vi "OAT FIR Preprocess Filter (N Channels).vi"(0 "scaled signals [EU]":waveform(dbl)[](array[waveform]), 1 "filter type":T3(ring), 2 "reset? (F)":bool, 5 "freq specs [Hz]":T2={"fpass 1"=100.0, "fstop 1"=200.0, "fpass 2"=0.0, "fstop 2"=0.0} {"fstop 2" format="%#.2f"; "fpass 2" format="%#.3f"; "fstop 1" format="%#.2f"; "fpass 1" format="%#.3f"}, 7 "ripple specs [dB]":T1={"passband ripple"=0.1, "stopband attenuation"=60.0} {"stopband attenuation" format="%#.2f"; "passband ripple" format="%#.2f"}, 11 "error in (no error)":errorcluster) -> (4 "filtered scaled signals [EU]":waveform(dbl)[](array[waveform]), 8 "taps":i32, 15 "error out":errorcluster)   [LabVIEW 2017, in "SoundVib_RefDataProcess.lvlib"]
doc: "Designs an FIR filter and filters the <B>scaled signal [EU]</B>. Wire data to the <B>scaled signal [EU]</B> input to determine the polymorphic instance to use or manually select the instance."
uses:
  <vilib>/addons/Sound and Vibration/Order Analysis/Referece Data Processing/SoundVib_RefDataProcess.lvlib
  <vilib>/addons/_NISVFA/_Shared subVIs/Common/svc_Check for Waveform Parameter Continuity (no state).vi
  <vilib>/addons/_NISVFA/_Shared subVIs/Common/svc_Get SV Channel Info.vi
  <vilib>/addons/_NISVFA/_Shared subVIs/Common/svc_Engineering Units to Unit Label.vi
  <vilib>/addons/_NISVFA/_Shared subVIs/Common/svc_Unit Label to Engineering Units.vi
  <vilib>/measure/NI_MAPro.lvlib
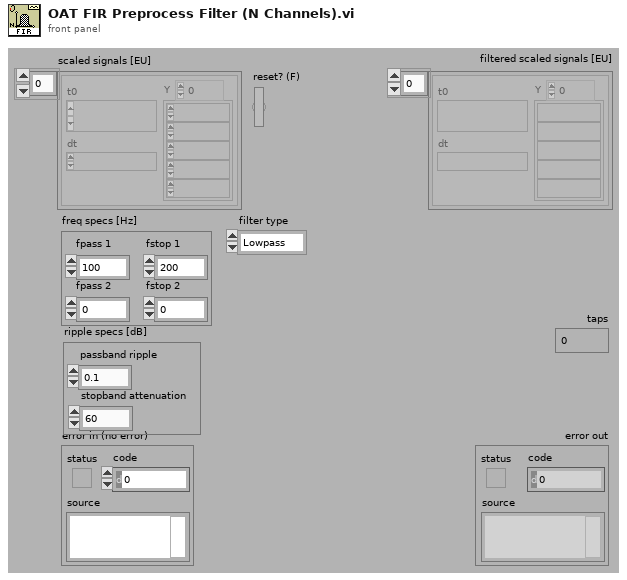
[diagram p1: front panel]
types:
  T1 = cluster{"passband ripple":dbl, "stopband attenuation":dbl}
  T2 = cluster{"fpass 1":dbl, "fstop 1":dbl, "fpass 2":dbl, "fstop 2":dbl}
  T3 = enum32{"Lowpass", "Highpass", "Bandpass", "Bandstop"}
  T4 = cluster{"dt equal":bool, "array length equal":bool, "number channels change":bool}
  T5 = cluster{"dt":bool, "t0 continuity":bool, "array length":bool, "channel info":bool, "name":bool}
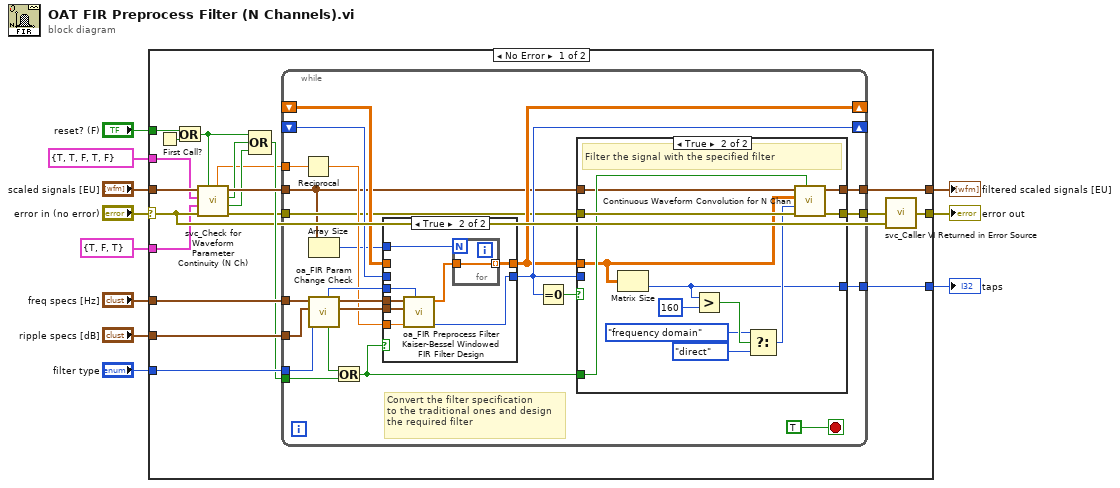
[diagram p0: block diagram]
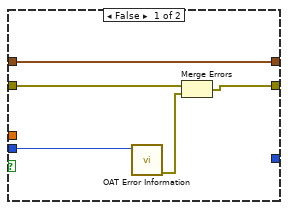
[diagram p3: hidden frame]
diagram:
  n1 = case shown="No Error" "error in (no error)" {
    selector: "error in (no error)" -> [w16 w83]
    tunnel: [w14 w83] -> w11
    tunnel: "scaled signals [EU]" -> [w25 w84]
    tunnel: "freq specs [Hz]" -> [w31 _]
    tunnel: "ripple specs [dB]" -> [w30 _]
    tunnel: "filter type" -> [w29 _]
    tunnel: [w28 w84] -> w7
    tunnel: [w27 _] -> w6
    tunnel: "reset? (F)" -> [w19 _]
    tunnel: T5 {"dt"=TRUE, "t0 continuity"=TRUE, "array length"=FALSE, "channel info"=TRUE, "name"=FALSE} ("checks for channel parameter change") -> [w13 _]
    tunnel: T4 {"dt equal"=TRUE, "array length equal"=FALSE, "number channels change"=TRUE} ("checks for multichannel parameters") -> [w12 _]
    frame No Error {
      n2 = First Call?() -> (First Call?: T/F=w26:bool)
      n3 = Or(x=w19, y=w26) -> (x .or. y?=w21:bool)
      n4 = call <vilib>:"svc_Check for Waveform Parameter Continuity (N Ch).vi"("restart averaging (F)"=w21, "error in (no error)"=w16, "checks for multichannel parameters"=w12, "checks for channel parameter change"=w13, "scaled signal(s)"=w25) -> ("error out"=w18:errorcluster, "multichannel parameter changed"=w22:bool, "waveform parameter changed"=w23:bool, "dup scaled signal(s)"=w24:waveform(dbl)[], "dt"=w15:dbl)  [unwired: 2 out]
      n5 = Compound Arithmetic op=OR(w21, w23, w22) -> (w20:bool)
      n6 = while {
        tunnel: [w43] -> w17
        tunnel: w31 -> [w50]
        tunnel: w30 -> [w49]
        tunnel: w29 -> [w48]
        tunnel: w24 -> [w33]
        shift-right: [w40] -> _
        shift-left: _ -> [w45]
        shift-right: [w42] -> _
        shift-left: _ -> [w44]
        tunnel: [w41] -> w28
        tunnel: [w35] -> w27
        tunnel: w20 -> [w39]
        tunnel: w18 -> [w37]
        tunnel: w15 -> [w34]
        stop <- TRUE stop-if-true
        # "Convert the filter specification\nto the traditional ones and design\nthe required filter"
        n7 = Reciprocal(x=w34) -> (1/x=w38:dbl)
        n8 = Array Size(array=w33) -> (size(s)=w32:i32)
        n9 = call <vilib>:"oa_FIR Param Change Check.vi"("filter type in"=w48, "ripple specs in [dB]"=w49, "freq specs in [Hz]"=w50) -> ("ripple specs out [dB]"=w53:cluster{"pass band":dbl, "stop band":dbl}, "freq specs out [Hz]"=w54:T2, "chang?"=w51:bool, "filter type out"=w52:T3)  [unwired: 4 in, 1 out]
        n10 = Or(x=w51, y=w39) -> (x .or. y?=w36:bool)
        n11 = case shown="True" w36 {
          tunnel: [w55 w61] -> w42
          tunnel: [w56 w58] -> w40
          tunnel: w45 -> [w56 _]
          tunnel: w44 -> [w55 _]
          tunnel: w54 -> [_ w64]
          tunnel: w53 -> [_ w63]
          tunnel: w52 -> [_ w60]
          tunnel: w38 -> [_ w62]
          tunnel: w32 -> [_ w57]
          frame False {
          }
          frame True {
            n12 = call <vilib>:"oa_FIR Preprocess Filter Kaiser-Bessel Windowed FIR Filter Design.vi"("filter types"=w60, "fs [Hz]"=w62, "ripple specs [dB]"=w63, "freq specs [Hz]"=w64) -> ("error"=w61:i32, "FIR Windowed Coefficients"=w59:dbl[])  [unwired: 6 in]
            n13 = for {
              N: w57 -> [_]
              tunnel: w59 -> [w65]
              tunnel: [w65] -> w58 mode=indexing
            }
          }
        }
        n14 = Equal To 0?(x=w42) -> (x = 0?=w46:bool)
        n15 = case shown="True" w46 {
          tunnel: w33 -> [w70 w73]
          tunnel: w36 -> [_ w75]
          tunnel: w40 -> [_ w72]
          tunnel: w42 -> [w69 _]
          tunnel: [w66 w76] -> w43
          tunnel: [w70 w77] -> w41
          tunnel: w37 -> [w68 w82]
          tunnel: [_ w71] -> w35
          frame False {
            n16 = call <vilib>:"OAT Error Information.vi"("error code"=w69) -> ("error out"=w67:errorcluster)  [unwired: 6 in]
            n17 = Merge Errors(w68, w67) -> (w66:errorcluster)
          }
          frame True {
            # "Filter the signal with the specified filter"
            n18 = Matrix Size(0:w72) -> (2:w71:i32)  [unwired: 1 out]
            n19 = Greater?(x=w71, y=160) -> (0:w80:bool)
            n20 = Select(t=enum32{"direct", "frequency domain"}."frequency domain" ("algorithm"), s=w80, f=enum32{"direct", "frequency domain"}."direct" ("algorithm")) -> (s? t:f=w74:enum32{"direct", "frequency domain"})
            n21 = call <vilib>:"Continuous Waveform Convolution for N Chan.vi"("reset"=w75, "error in (no error)"=w82, "algorithm"=w74, "kernels"=w72, "signals in"=w73) -> ("error out"=w76:errorcluster, "signals out"=w77:waveform(dbl)[])  [unwired: 5 in]
          }
        }
      }
      n22 = call <vilib>:"svc_Caller VI Returned in Error Source.vi"("warning input to caller"=w16, "error in (no error)"=w17) -> ("error out"=w14:errorcluster)  [unwired: 3 in]
    }
    frame Error {
    }
  }
  "error out" <- w11
  "filtered scaled signals [EU]" <- w7
  "taps" <- w6
